vi "Callback Change Channel Name.vi"(6 "Variant":variant, 8 "error in (no error)":errorcluster, 9 "Old Values":string[][](array[string]), 10 "object ref in":T1, 11 "Table Change":T2) -> (0 "error out":errorcluster)   [LabVIEW 2015, in "PID Module editor node.lvclass"]
doc: "This VI gets called automatically when changes are made to the 'Name' column of the table and must handle changes appropriately. Register this callback using the appropriate 'Define Column' VI from the Table API."
uses:
  PID Module editor node.lvclass
  <vilib>/NI/DCAF/Tag Editor Core/Table API/Table Manager/Cell Change.ctl
  <vilib>/NI/DCAF/Tag Editor Core/Table API/Table Manager/object ref.ctl
  <vilib>/NI/DCAF/Tag Editor Core/Configuration Editor/Classes/Engine Parent/Engine Parent Editor Node.lvclass
  <vilib>/NI/DCAF/Tag Editor Core/Configuration Editor/Classes/Module editor node/module editor node.lvclass
  module/configuration/PID Module configuration.lvclass
  module/configuration/PID Module configuration.lvclass/PID Module configuration.ctl
  module/configuration/Get Line Name.vi
  <vilib>/NI/Tag Bus Module Framework/module configuration/FindDuplicate.vi
  <vilib>/Utility/error.llb/Error Cluster From Error Code.vi
  <vilib>/NI/Tag Bus Module Framework/channel/TBM channel.lvclass
  <vilib>/NI/Tag Bus/tag/tag descriptor.lvclass
  <vilib>/NI/Configuration Framework/serializable configuration/NISE_CEF_serializable configuration.lvclass
  <vilib>/NI/Module Execution Interface/Engine Configuration/engine configuration.lvclass
  <vilib>/NI/DCAF/Tag Editor Core/Table API/Table Manager.lvlib
  <vilib>/NI/DCAF/Tag Editor Core/Table API/Table Manager/Table Manager.lvclass
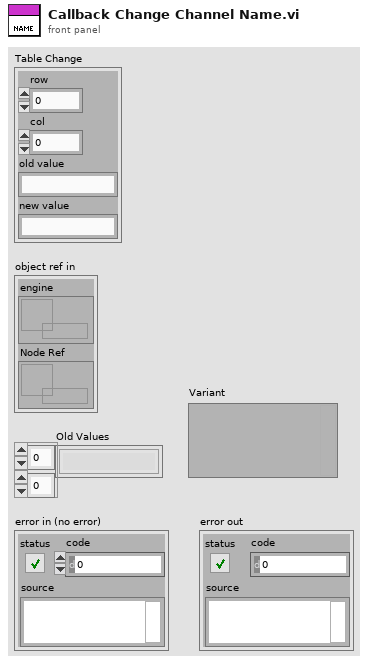
[diagram p1: front panel]
types:
  T1 = typedef "Table Manager.lvlib/Table Manager.lvclass/object ref.ctl" = cluster{"engine":refnum<data-value>, "Node Ref":refnum<data-value>}
  T2 = typedef "Table Manager.lvlib/Cell Change.ctl" = cluster{"row":i32, "col":i32, "old value":string, "new value":string}
  T3 = typedef "PID Module configuration.lvclass/Line.ctl" = cluster{"PID ID":string, "Setpoint":refnum<class "TBM channel.lvclass">, "Variable":refnum<class "TBM channel.lvclass">, "Output":refnum<class "TBM channel.lvclass">, "Output High":refnum<class "TBM channel.lvclass">, "Output Low":refnum<class "TBM channel.lvclass">, "P":refnum<class "TBM channel.lvclass">, "I":refnum<class "TBM channel.lvclass">, "D":refnum<class "TBM channel.lvclass">}
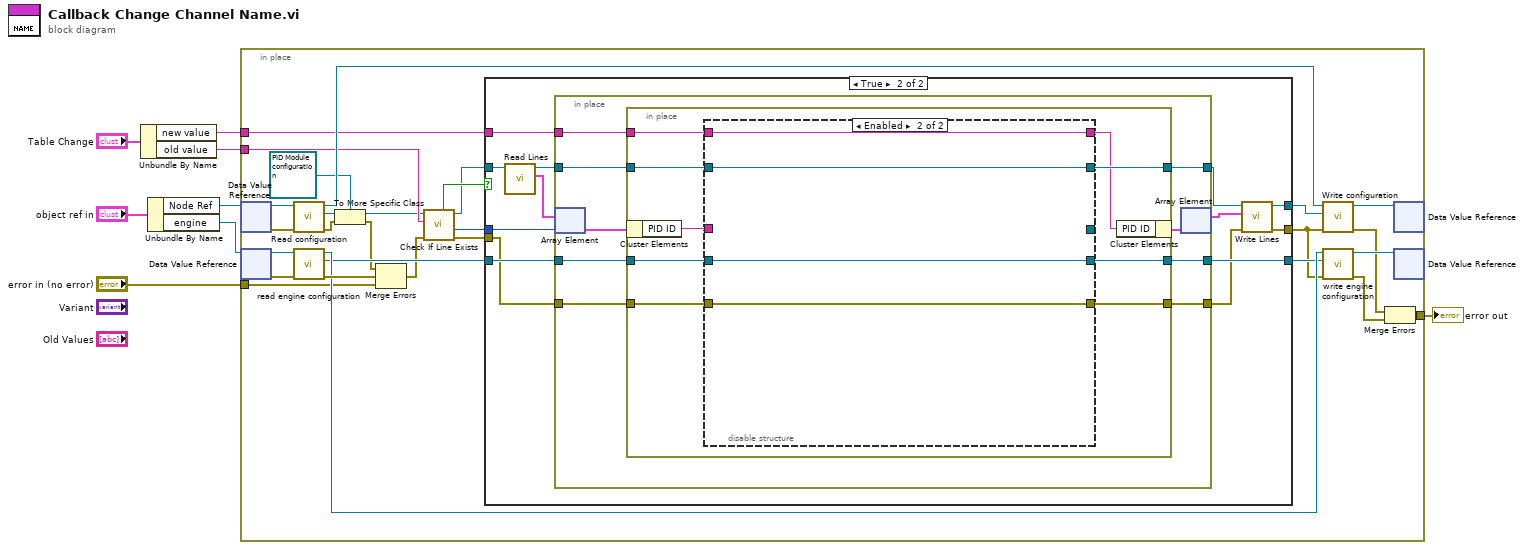
[diagram p0: block diagram]
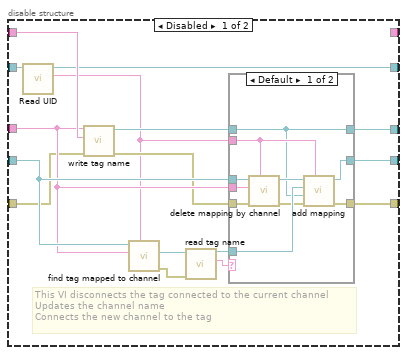
[diagram p3: hidden frame]
diagram:
  n1 = Unbundle By Name("Table Change") -> ("new value"=w1:string, "old value"=w2:string)
  n2 = Unbundle By Name("object ref in") -> ("Node Ref"=w5:refnum<data-value>, "engine"=w4:refnum<data-value>)
  n3 = in-place {
    in-place-border: [w29] -> w8
    in-place-border: "error in (no error)" -> [w25]
    in-place-border: w2 -> [w23]
    in-place-border: w1 -> [w20]
    n4 = in-place-dvr #1(w5) -> (w18:refnum<class "module editor node.lvclass">, w28:errorcluster)
    n5 = in-place-dvr #2(w4) -> (w36:refnum<class "Engine Parent Editor Node.lvclass">, w37:errorcluster)
    n6 = call-dynamic "Read configuration.vi"("error in"=w28, "NISE_CEF_serializable node in"=w18) -> ("error out"=w10:errorcluster, "configuration"=w26:refnum<class "NISE_CEF_serializable configuration.lvclass">, "NISE_CEF_serializable node out"=w27:refnum<class "module editor node.lvclass">)  [unwired: 7 in]
    n7 = call <vilib>:"read engine configuration.vi"("error in"=w37, "Engine Parent Editor Node in"=w36) -> ("error out"=w33:errorcluster, "engine configuration"=w15:refnum<class "engine configuration.lvclass">, "Engine Parent Editor Node out"=w32:refnum<class "Engine Parent Editor Node.lvclass">)  [unwired: 7 in]
    n8 = To More Specific Class(target class=refnum<class "PID Module configuration.lvclass"> refnum ("tag bus configurable plugin module configuration"), reference=w26, error in=w10) -> (specific class reference=w17:refnum<class "PID Module configuration.lvclass">, error out=w9:errorcluster)
    n9 = Merge Errors(w9, w33, w25) -> (w13:errorcluster)
    n10 = call-dynamic "Check If Line Exists.vi"("error in"=w13, "Name to Locate"=w23, "PID Module configuration in"=w17) -> ("error out"=w14:errorcluster, "Index"=w21:i32, "PID Module configuration out"=w12:refnum<class "PID Module configuration.lvclass">, "Found?"=w19:bool)  [unwired: 4 in, 1 out]
    n11 = case shown="True" w19 {
      tunnel: [w40 w53] -> w22
      tunnel: w12 -> [w40 w52]
      tunnel: w21 -> [_ w49]
      tunnel: w20 -> [_ w48]
      tunnel: w15 -> [w39 w47]
      tunnel: [w39 w46] -> w16
      tunnel: [w38 w45] -> w11
      tunnel: w14 -> [w38 w43]
      frame False {
      }
      frame True {
        n12 = call "Read Lines.vi"("PID Module configuration in"=w52) -> ("Lines"=w51:T3[], "PID Module configuration out"=w42:refnum<class "PID Module configuration.lvclass">)  [unwired: 8 in, 1 out]
        n13 = in-place {
          in-place-border: w48 -> [w60]
          in-place-border: w47 -> [w59]
          in-place-border: [w58] -> w46
          in-place-border: [w57] -> w44
          in-place-border: w43 -> [w56]
          in-place-border: w42 -> [w55]
          in-place-border: [w54] -> w41
          n14 = in-place-array #3(w51, w49) -> (w62:T3)
          n15 = in-place {
            in-place-border: w60 -> [w71]
            in-place-border: w59 -> [w69]
            in-place-border: [w70] -> w58
            in-place-border: [w66] -> w57
            in-place-border: w56 -> [w67]
            in-place-border: w55 -> [w65]
            in-place-border: [w64] -> w54
            n16 = in-place-cluster #4(w62) -> ("PID ID"=w68:string)
            n17 = disable-structure shown="Enabled" {
              disable-tunnel: w71 -> [w87 w104]
              disable-tunnel: [w86 w102] -> w70
              disable-tunnel: w69 -> [w85 w102]
              disable-tunnel: w68 -> [w84 _]
              disable-tunnel: w67 -> [w79 w101]
              disable-tunnel: [w77 w101] -> w66
              disable-tunnel: w65 -> [w75 w103]
              disable-tunnel: [w74 w103] -> w64
              disable-tunnel: [w73 _] -> _
              disable-tunnel: [_ w104] -> w63
              frame Disabled {
                # "This VI disconnects the tag connected to the current channel\nUpdates the channel name\nConnects the new channel to the tag"
                n18 = call <vilib>:"Read UID.vi"("configuration in"=w75) -> ("instance id"=w76:string, "configuration out"=w74:refnum<class "PID Module configuration.lvclass">)  [unwired: 8 in, 1 out]
                n19 = call <vilib>:"write tag name.vi"("error in"=w79, "name"=w87, "system tag in"=w84) -> ("error out"=w78:errorcluster, "system tag out"=w80:refnum<class "tag descriptor.lvclass">)  [unwired: 7 in]
                n20 = call <vilib>:"find tag mapped to channel.vi"("owner"=w76, "channel"=w84, "engine configuration in"=w85) -> ("error out"=w72:errorcluster, "tag"=w83:refnum<class "tag descriptor.lvclass">)  [unwired: 6 in, 1 out]
                n21 = call <vilib>:"read tag name.vi"("error in"=w72, "system tag in"=w83) -> ("name"=w82:string, "system tag out"=w81:refnum<class "tag descriptor.lvclass">)  [unwired: 7 in, 1 out]
                n22 = case shown="Default" w82 {
                  tunnel: [w96 w100] -> w86
                  tunnel: w85 -> [w95 w100]
                  tunnel: w76 -> [w94 _]
                  tunnel: w84 -> [w93 _]
                  tunnel: w81 -> [w92 _]
                  tunnel: w80 -> [w88 w98]
                  tunnel: [w90 w99] -> w77
                  tunnel: w78 -> [w89 w99]
                  tunnel: [w88 w98] -> w73
                  frame Default {
                    n23 = call <vilib>:"delete mapping by channel.vi"("owner ID"=w94, "error in"=w89, "channel"=w93, "engine configuration in"=w95) -> ("error out"=w91:errorcluster, "engine configuration out"=w97:refnum<class "engine configuration.lvclass">)  [unwired: 6 in]
                    n24 = call-dynamic "add mapping.vi"("owner ID"=w94, "error in"=w91, "channel"=w88, "tag descriptor"=w92, "engine configuration"=w97) -> ("error out"=w90:errorcluster, "engine configuration out"=w96:refnum<class "engine configuration.lvclass">)  [unwired: 5 in]
                  }
                  frame "" {
                  }
                }
              }
              frame Enabled {
              }
            }
            n25 = in-place-cluster #4("PID ID"=w63) -> (w61:T3)
          }
          n26 = in-place-array #3(w61) -> (w50:T3[])  [unwired: 1 out]
        }
        n27 = call "Write Lines.vi"("error in (no error)"=w44, "Lines"=w50, "PID Module configuration in"=w41) -> ("error out"=w45:errorcluster, "PID Module configuration out"=w53:refnum<class "PID Module configuration.lvclass">)  [unwired: 7 in]
      }
    }
    n28 = call-dynamic "Write configuration.vi"("error in"=w11, "configuration"=w22, "NISE_CEF_serializable node in"=w27) -> ("error out"=w30:errorcluster, "NISE_CEF_serializable node out"=w34:refnum<class "module editor node.lvclass">)  [unwired: 7 in]
    n29 = call <vilib>:"write engine configuration.vi"("error in"=w11, "engine configuration"=w16, "Engine Parent Editor Node in"=w32) -> ("error out"=w31:errorcluster, "Engine Parent Editor Node out"=w35:refnum<class "Engine Parent Editor Node.lvclass">)  [unwired: 7 in]
    n30 = Merge Errors(w30, w31) -> (w29:errorcluster)
    n31 = in-place-dvr #1(w34) -> ()  [unwired: 2 out]
    n32 = in-place-dvr #2(w35) -> ()  [unwired: 2 out]
  }
  "error out" <- w8
